vi "Mqtt_Msg_Decode.vi"(8 "error in (no error)":errorcluster, 11 "CMD_Response":string="{\n    \"ID\": \"ac0cc47e-6714-46c6-9d0a-105aa9849fbe\",\n    \"TO\": \"9C6B00576F17\",\n    \"FROM\": \"6805CAB81F91\",\n    \"CMD\": 3,\n    \"CONTENT\": [\n      {\n        \"RACK\": \"101\",\n        \"DUT\": \"1\",\n        \"STATUS\": \"READY\", //READY, MAINTAIN, CLOSE\n        \"REQ_ID\": \"9c67a4e5-71cc-4fd4-b3a2-c356c70535d5\"\n      }\n    ],\n    \"STATUS\": true,\n    \"ERRCODE\": \"\",\n    \"ERRMSG\": \"\",\n    \"TIMESTAMP\": 1757865617\n  }") -> (0 "error out":errorcluster, 3 "Result":T1)   [LabVIEW 2020]
uses:
  <vilib>/addons/JSON API/JSON Value/JSON Value.lvclass
  Ctrl/ReplyCMD0.ctl
  Ctrl/ReplyCMD3.ctl
  Ctrl/ReplyCMD6.ctl
  Ctrl/ReplyCMD9.ctl
  Ctrl/ReplyCMD23.ctl
  Ctrl/ReplyCMD24.ctl
  Ctrl/ReplyCMD25.ctl
  <vilib>/addons/JSON API/JSON Value/Set from JSON string.vi
  <vilib>/addons/JSON API/JSON Value/Get as JSON string.vi
  <vilib>/addons/JSON API/JSON Scalar/Get as U32.vi
  <vilib>/addons/JSON API/JSON Scalar/Get as Boolean.vi
  <vilib>/addons/JSON API/JSON Scalar/Get as Text.vi
  <vilib>/addons/JSON API/JSON Value/Get Array by name.vi
  <vilib>/addons/JSON API/JSON Value/Get Item by name array.vi
  <vilib>/addons/JSON API/Get Polymorphic/JSON GetSet.lvlib
  <vilib>/addons/_JKI.lib/Serialization/JSON/JKI JSON Serialization.lvlib
  <vilib>/addons/JSON API/JSON Scalar/JSON Scalar.lvclass
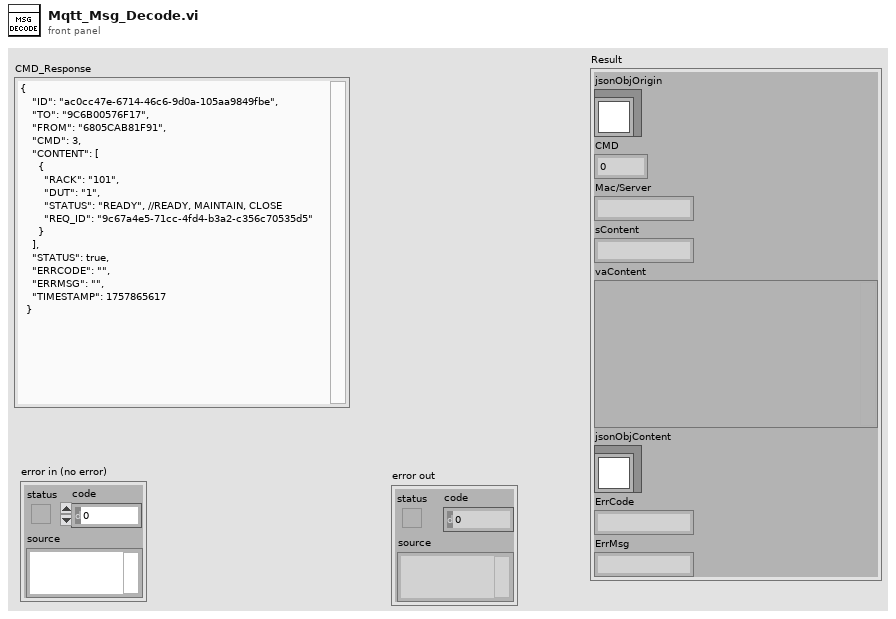
[diagram p1: front panel]
types:
  T1 = cluster{"jsonObjOrigin":refnum<class "JSON Value.lvclass">, "CMD":u32, "Mac/Server":string, "sContent":string, "vaContent":variant, "jsonObjContent":refnum<class "JSON Value.lvclass">, "ErrCode":string, "ErrMsg":string}
  T2 = typedef "ReplyCMD0.ctl" = cluster{"ADD_TOPIC":string}
  T3 = typedef "ReplyCMD3.ctl" = cluster{"RACK":string, "DUT":string, "STATUS":string}
  T4 = typedef "ReplyCMD6.ctl" = cluster{"STATION":string, "RACK":string, "SN":string, "RESULT":string}
  T5 = typedef "ReplyCMD9.ctl" = cluster{"RACK":string, "DUT":string, "CMD":string}
  T6 = typedef "ReplyCMD23.ctl" = cluster{"STATION":string, "RACK":string, "DUT":string, "SN":string, "DESC":string, "RESULT":string, "SET_RACK_STATUS":string}
  T7 = typedef "ReplyCMD24.ctl" = cluster{"STATION":string, "RACK":string, "DUT":string, "SN":string, "MAC_BMC":string, "MAC_SWITCH":string, "MAC_SCM":string}
  T8 = typedef "ReplyCMD25.ctl" = cluster{"STATION":string, "RACK":u32, "DUT":u32}
  T9 = cluster{"H/P":cluster{"Rack#":string, "DUT Status":string[]}[], "F/T-B":cluster{"Rack#":string, "DUT Status":string[]}[], "F/T":cluster{"Rack#":string, "DUT Status":string[]}[]}
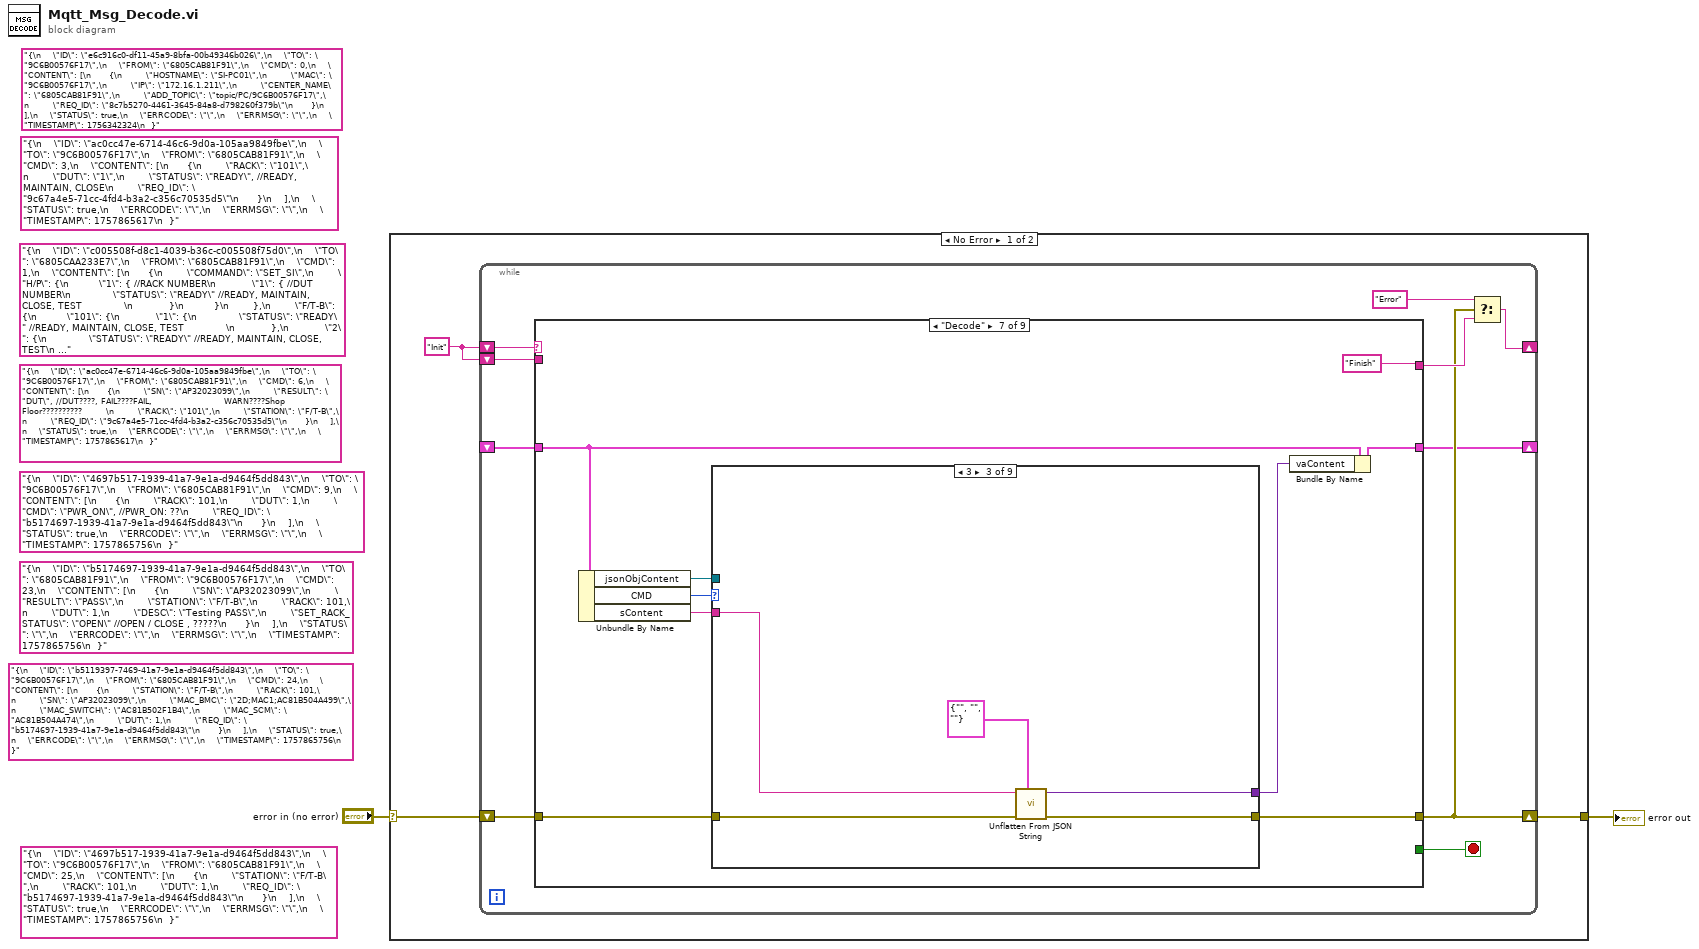
[diagram p0: block diagram]
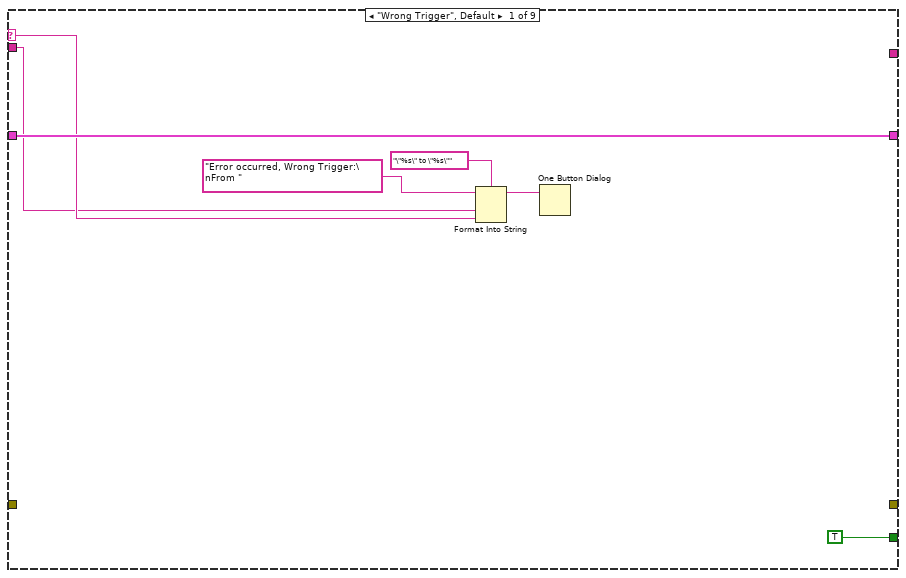
[diagram p2: hidden frame]
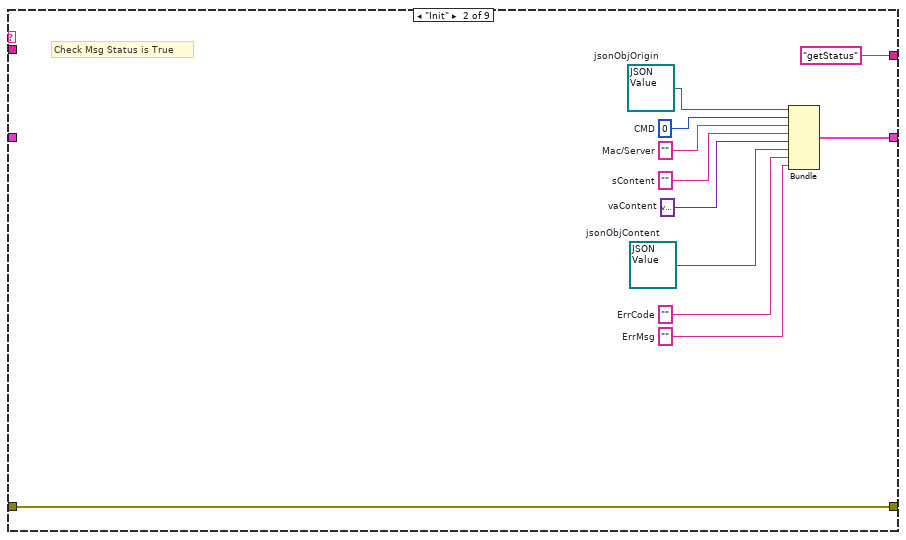
[diagram p3: hidden frame]
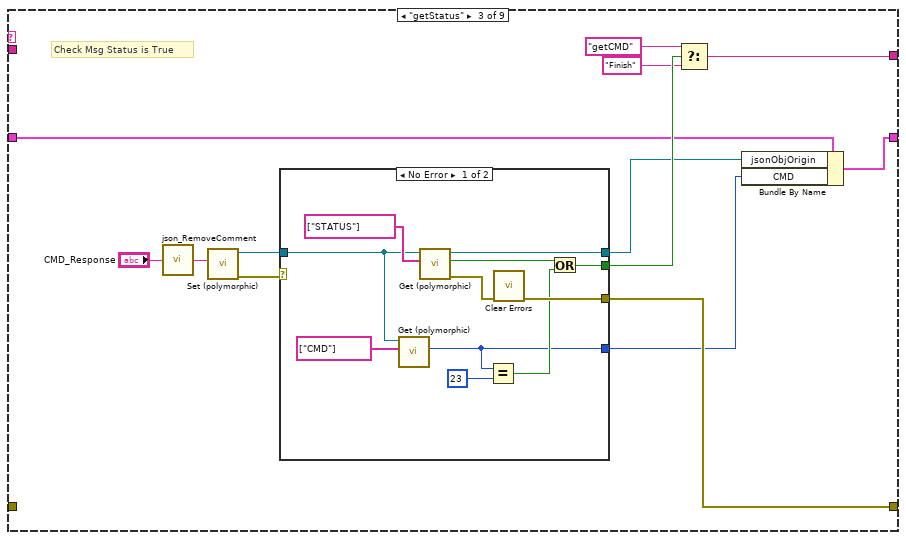
[diagram p4: hidden frame]
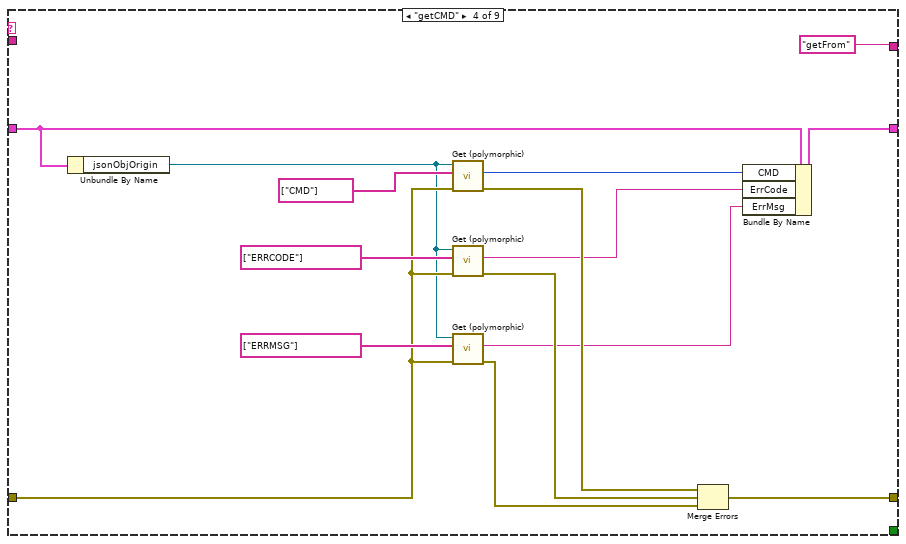
[diagram p6: hidden frame]
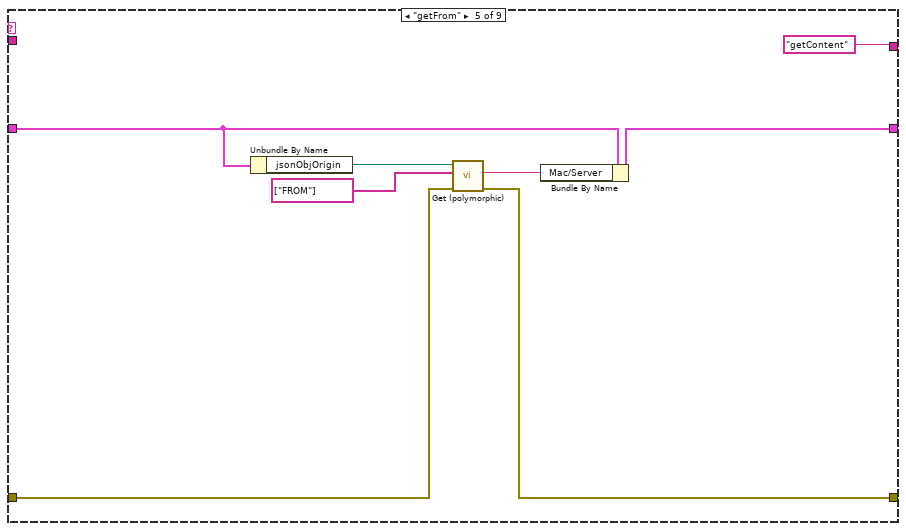
[diagram p7: hidden frame]
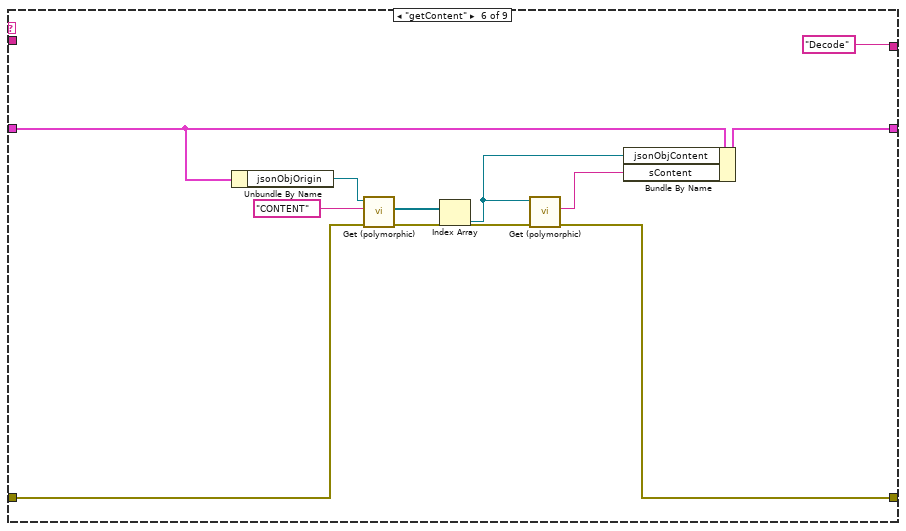
[diagram p8: hidden frame]
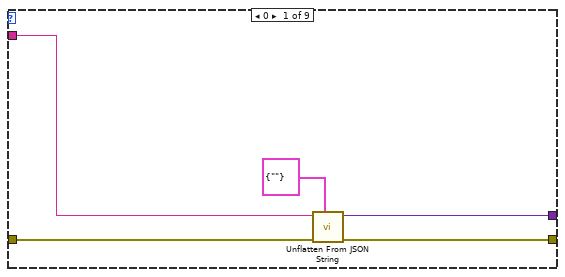
[diagram p9: hidden frame]
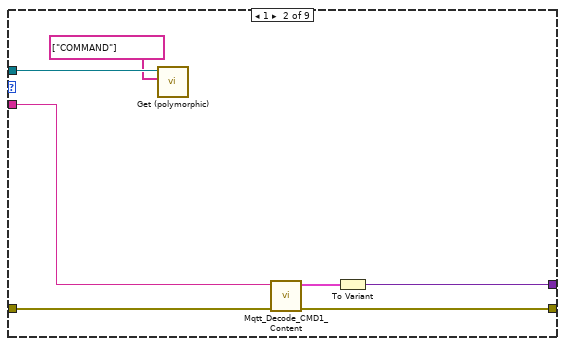
[diagram p10: hidden frame]
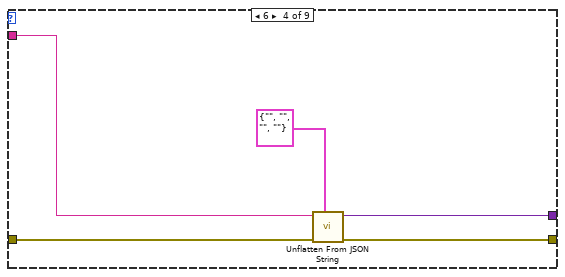
[diagram p11: hidden frame]
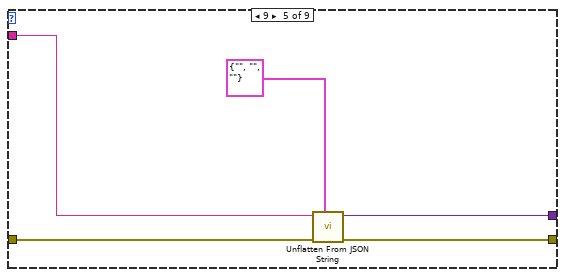
[diagram p12: hidden frame]
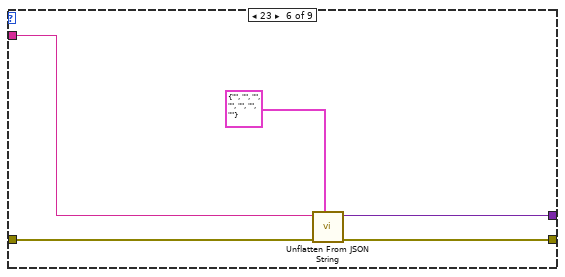
[diagram p13: hidden frame]
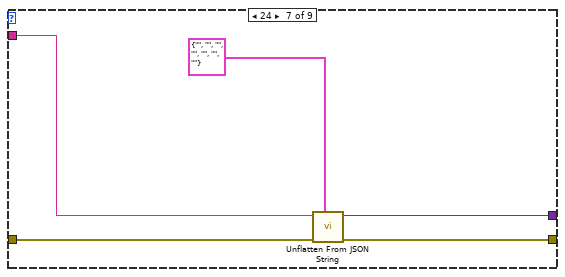
[diagram p14: hidden frame]
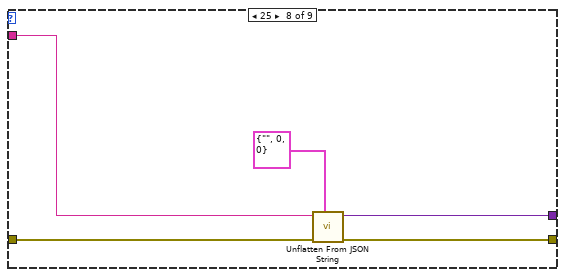
[diagram p15: hidden frame]
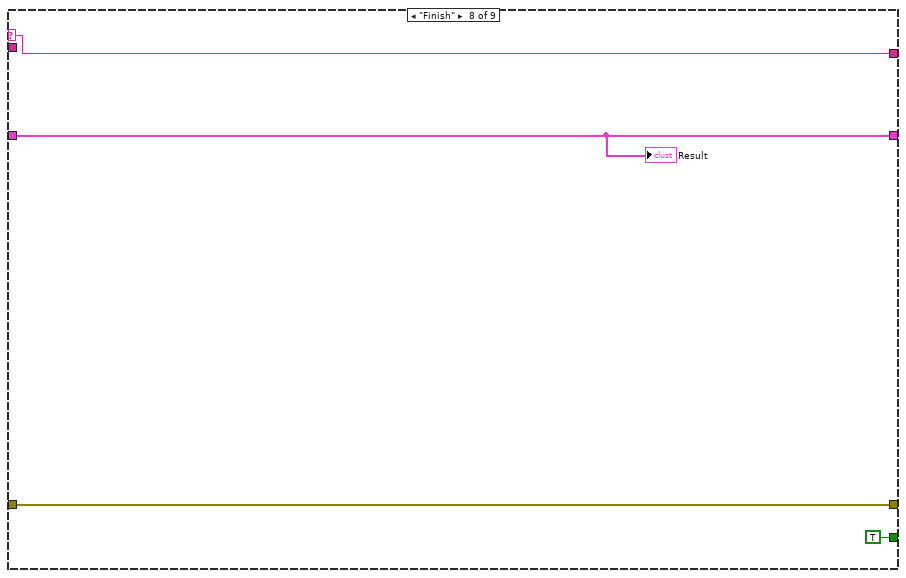
[diagram p17: hidden frame]
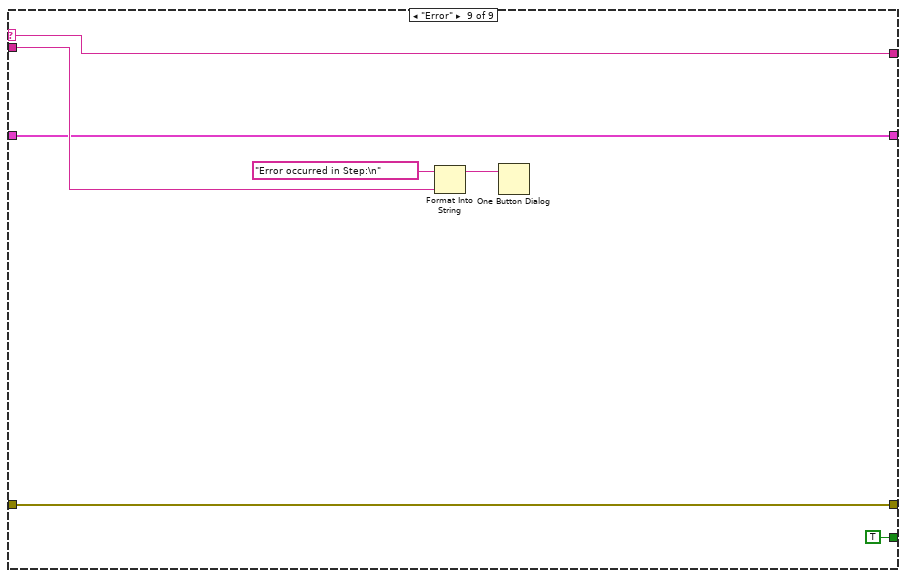
[diagram p18: hidden frame]
diagram:
  (unwired) "{\n    \"ID\": \"b5119397-7469-41a7-9e1a-d9464f5dd843\",\n    \"TO\": \"9C6B00576F17\",\n    \"FROM\": \"6805CAB81F91\",\n    \"CMD\": 24,\n    \"CONTENT\": [\n      {\n        \"STATION\": \"F/T-B\",\n        \"RACK\": 101,\n        \"SN\": \"AP32023099\",\n        \"MAC_BMC\": \"2D;MAC1;AC81B504A499\",\n        \"MAC_SWITCH\": \"AC81B502F1B4\",\n        \"MAC_SCM\": \"AC81B504A474\",\n        \"DUT\": 1,\n        \"REQ_ID\": \"b5174697-1939-41a7-9e1a-d9464f5dd843\"\n      }\n    ],\n    \"STATUS\": true,\n    \"ERRCODE\": \"\",\n    \"ERRMSG\": \"\",\n    \"TIMESTAMP\": 1757865756\n  }" ("CMD_Response")
  (unwired) "{\n    \"ID\": \"b5174697-1939-41a7-9e1a-d9464f5dd843\",\n    \"TO\": \"6805CAB81F91\",\n    \"FROM\": \"9C6B00576F17\",\n    \"CMD\": 23,\n    \"CONTENT\": [\n      {\n        \"SN\": \"AP32023099\",\n        \"RESULT\": \"PASS\",\n        \"STATION\": \"F/T-B\",\n        \"RACK\": 101,\n        \"DUT\": 1,\n        \"DESC\": \"Testing PASS\",\n        \"SET_RACK_STATUS\": \"OPEN\" //OPEN / CLOSE , ?????\n      }\n    ],\n    \"STATUS\": \"\",\n    \"ERRCODE\": \"\",\n    \"ERRMSG\": \"\",\n    \"TIMESTAMP\": 1757865756\n  }" ("CMD_Response")
  (unwired) "{\n    \"ID\": \"4697b517-1939-41a7-9e1a-d9464f5dd843\",\n    \"TO\": \"9C6B00576F17\",\n    \"FROM\": \"6805CAB81F91\",\n    \"CMD\": 9,\n    \"CONTENT\": [\n      {\n        \"RACK\": 101,\n        \"DUT\": 1,\n        \"CMD\": \"PWR_ON\", //PWR_ON: ??\n        \"REQ_ID\": \"b5174697-1939-41a7-9e1a-d9464f5dd843\"\n      }\n    ],\n    \"STATUS\": true,\n    \"ERRCODE\": \"\",\n    \"ERRMSG\": \"\",\n    \"TIMESTAMP\": 1757865756\n  }" ("CMD_Response")
  (unwired) "{\n    \"ID\": \"ac0cc47e-6714-46c6-9d0a-105aa9849fbe\",\n    \"TO\": \"9C6B00576F17\",\n    \"FROM\": \"6805CAB81F91\",\n    \"CMD\": 6,\n    \"CONTENT\": [\n      {\n        \"SN\": \"AP32023099\",\n        \"RESULT\": \"DUT\", //DUT????, FAIL????FAIL,                        WARN????Shop Floor??????????        \n        \"RACK\": \"101\",\n        \"STATION\": \"F/T-B\",\n        \"REQ_ID\": \"9c67a4e5-71cc-4fd4-b3a2-c356c70535d5\"\n      }\n    ],\n    \"STATUS\": true,\n    \"ERRCODE\": \"\",\n    \"ERRMSG\": \"\",\n    \"TIMESTAMP\": 1757865617\n  }" ("CMD_Response")
  (unwired) "{\n    \"ID\": \"c005508f-d8c1-4039-b36c-c005508f75d0\",\n    \"TO\": \"6805CAA233E7\",\n    \"FROM\": \"6805CAB81F91\",\n    \"CMD\": 1,\n    \"CONTENT\": [\n      {\n        \"COMMAND\": \"SET_SI\",\n        \"H/P\": {\n          \"1\": { //RACK NUMBER\n            \"1\": { //DUT NUMBER\n              \"STATUS\": \"READY\" //READY, MAINTAIN, CLOSE, TEST              \n            }\n          }\n        },\n        \"F/T-B\": {\n          \"101\": {\n            \"1\": {\n              \"STATUS\": \"READY\" //READY, MAINTAIN, CLOSE, TEST              \n            },\n            \"2\": {\n              \"STATUS\": \"READY\" //READY, MAINTAIN, CLOSE, TEST\n            },\n            \"3\": {\n              \"STATUS\": \"READY\" //READY, MAINTAIN, CLOSE, TEST\n            },\n            \"4\": {\n              \"STATUS\": \"READY\" //READY, MAINTAIN, CLOSE, TEST\n            },\n            \"5\": {\n              \"STATUS\": \"READY\" //READY, MAINTAIN, CLOSE, TEST\n            }\n          },\n          \"102\": {\n            \"1\": {\n              \"STATUS\": \"READY\" //READY, MAINTAIN, CLOSE, TEST              \n            },\n            \"2\": {\n              \"STATUS\": \"READY\" //READY, MAINTAIN, CLOSE, TEST\n            },\n            \"3\": {\n              \"STATUS\": \"READY\" //READY, MAINTAIN, CLOSE, TEST\n            },\n            \"4\": {\n              \"STATUS\": \"READY\" //READY, MAINTAIN, CLOSE, TEST\n            },\n            \"5\": {\n              \"STATUS\": \"READY\" //READY, MAINTAIN, CLOSE, TEST\n            }\n          },\n          \"103\": {\n            \"1\": {\n              \"STATUS\": \"READY\" //READY, MAINTAIN, CLOSE, TEST              \n            },\n            \"2\": {\n              \"STATUS\": \"READY\" //READY, MAINTAIN, CLOSE, TEST\n            },\n            \"3\": {\n              \"STATUS\": \"READY\" //READY, MAINTAIN, CLOSE, TEST\n            },\n            \"4\": {\n              \"STATUS\": \"READY\" //READY, MAINTAIN, CLOSE, TEST\n            },\n            \"5\": {\n              \"STATUS\": \"READY\" //READY, MAINTAIN, CLOSE, TEST\n            }\n          },\n          \"104\": {\n            \"1\": {\n              \"STATUS\": \"READY\" //READY, MAINTAIN, CLOSE, TEST              \n            },\n            \"2\": {\n              \"STATUS\": \"READY\" //READY, MAINTAIN, CLOSE, TEST\n            },\n            \"3\": {\n              \"STATUS\": \"READY\" //READY, MAINTAIN, CLOSE, TEST\n            },\n            \"4\": {\n              \"STATUS\": \"READY\" //READY, MAINTAIN, CLOSE, TEST\n            },\n            \"5\": {\n              \"STATUS\": \"READY\" //READY, MAINTAIN, CLOSE, TEST\n            }\n          },\n          \"105\": {\n            \"1\": {\n              \"STATUS\": \"READY\" //READY, MAINTAIN, CLOSE, TEST              \n            },\n            \"2\": {\n              \"STATUS\": \"READY\" //READY, MAINTAIN, CLOSE, TEST\n            },\n            \"3\": {\n              \"STATUS\": \"READY\" //READY, MAINTAIN, CLOSE, TEST\n            },\n            \"4\": {\n              \"STATUS\": \"READY\" //READY, MAINTAIN, CLOSE, TEST\n            },\n            \"5\": {\n              \"STATUS\": \"READY\" //READY, MAINTAIN, CLOSE, TEST\n            }\n          },\n          \"106\": {\n            \"1\": {\n              \"STATUS\": \"READY\" //READY, MAINTAIN, CLOSE, TEST              \n            },\n            \"2\": {\n              \"STATUS\": \"READY\" //READY, MAINTAIN, CLOSE, TEST\n            },\n            \"3\": {\n              \"STATUS\": \"READY\" //READY, MAINTAIN, CLOSE, TEST\n            },\n            \"4\": {\n              \"STATUS\": \"READY\" //READY, MAINTAIN, CLOSE, TEST\n            },\n            \"5\": {\n              \"STATUS\": \"READY\" //READY, MAINTAIN, CLOSE, TEST\n            }\n          },\n          \"107\": {\n            \"1\": {\n              \"STATUS\": \"READY\" //READY, MAINTAIN, CLOSE, TEST              \n            },\n            \"2\": {\n              \"STATUS\": \"READY\" //READY, MAINTAIN, CLOSE, TEST\n            },\n            \"3\": {\n              \"STATUS\": \"READY\" //READY, MAINTAIN, CLOSE, TEST\n            },\n            \"4\": {\n              \"STATUS\": \"READY\" //READY, MAINTAIN, CLOSE, TEST\n            },\n            \"5\": {\n              \"STATUS\": \"READY\" //READY, MAINTAIN, CLOSE, TEST\n            }\n          },\n          \"108\": {\n            \"1\": {\n              \"STATUS\": \"READY\" //READY, MAINTAIN, CLOSE, TEST              \n            },\n            \"2\": {\n              \"STATUS\": \"READY\" //READY, MAINTAIN, CLOSE, TEST\n            },\n            \"3\": {\n              \"STATUS\": \"READY\" //READY, MAINTAIN, CLOSE, TEST\n            },\n            \"4\": {\n              \"STATUS\": \"READY\" //READY, MAINTAIN, CLOSE, TEST\n            },\n            \"5\": {\n              \"STATUS\": \"READY\" //READY, MAINTAIN, CLOSE, TEST\n            }\n          },\n          \"109\": {\n            \"1\": {\n              \"STATUS\": \"READY\" //READY, MAINTAIN, CLOSE, TEST              \n            },\n            \"2\": {\n              \"STATUS\": \"READY\" //READY, MAINTAIN, CLOSE, TEST\n            },\n            \"3\": {\n              \"STATUS\": \"READY\" //READY, MAINTAIN, CLOSE, TEST\n            },\n            \"4\": {\n              \"STATUS\": \"READY\" //READY, MAINTAIN, CLOSE, TEST\n            },\n            \"5\": {\n              \"STATUS\": \"READY\" //READY, MAINTAIN, CLOSE, TEST\n            }\n          },\n          \"110\": {\n            \"1\": {\n              \"STATUS\": \"READY\" //READY, MAINTAIN, CLOSE, TEST              \n            },\n            \"2\": {\n              \"STATUS\": \"READY\" //READY, MAINTAIN, CLOSE, TEST\n            },\n            \"3\": {\n              \"STATUS\": \"READY\" //READY, MAINTAIN, CLOSE, TEST\n            },\n            \"4\": {\n              \"STATUS\": \"READY\" //READY, MAINTAIN, CLOSE, TEST\n            },\n            \"5\": {\n              \"STATUS\": \"READY\" //READY, MAINTAIN, CLOSE, TEST\n            }\n          },\n          \"111\": {\n            \"1\": {\n              \"STATUS\": \"READY\" //READY, MAINTAIN, CLOSE, TEST              \n            },\n            \"2\": {\n              \"STATUS\": \"READY\" //READY, MAINTAIN, CLOSE, TEST\n            },\n            \"3\": {\n              \"STATUS\": \"READY\" //READY, MAINTAIN, CLOSE, TEST\n            },\n            \"4\": {\n              \"STATUS\": \"READY\" //READY, MAINTAIN, CLOSE, TEST\n            },\n            \"5\": {\n              \"STATUS\": \"READY\" //READY, MAINTAIN, CLOSE, TEST\n            }\n          },\n          \"112\": {\n            \"1\": {\n              \"STATUS\": \"READY\" //READY, MAINTAIN, CLOSE, TEST              \n            },\n            \"2\": {\n              \"STATUS\": \"READY\" //READY, MAINTAIN, CLOSE, TEST\n            },\n            \"3\": {\n              \"STATUS\": \"READY\" //READY, MAINTAIN, CLOSE, TEST\n            },\n            \"4\": {\n              \"STATUS\": \"READY\" //READY, MAINTAIN, CLOSE, TEST\n            },\n            \"5\": {\n              \"STATUS\": \"READY\" //READY, MAINTAIN, CLOSE, TEST\n            }\n          }\n        },\n        \"F/T\": {\n          \"201\": {\n            \"1\": {\n              \"STATUS\": \"READY\" //READY, MAINTAIN, CLOSE, TEST              \n            },\n            \"2\": {\n              \"STATUS\": \"READY\" //READY, MAINTAIN, CLOSE, TEST\n            },\n            \"3\": {\n              \"STATUS\": \"READY\" //READY, MAINTAIN, CLOSE, TEST\n            },\n            \"4\": {\n              \"STATUS\": \"READY\" //READY, MAINTAIN, CLOSE, TEST\n            },\n            \"5\": {\n              \"STATUS\": \"READY\" //READY, MAINTAIN, CLOSE, TEST\n            }\n          },\n          \"202\": {\n            \"1\": {\n              \"STATUS\": \"READY\" //READY, MAINTAIN, CLOSE, TEST              \n            },\n            \"2\": {\n              \"STATUS\": \"READY\" //READY, MAINTAIN, CLOSE, TEST\n            },\n            \"3\": {\n              \"STATUS\": \"READY\" //READY, MAINTAIN, CLOSE, TEST\n            },\n            \"4\": {\n              \"STATUS\": \"READY\" //READY, MAINTAIN, CLOSE, TEST\n            },\n            \"5\": {\n              \"STATUS\": \"READY\" //READY, MAINTAIN, CLOSE, TEST\n            }\n          },\n          \"203\": {\n            \"1\": {\n              \"STATUS\": \"READY\" //READY, MAINTAIN, CLOSE, TEST              \n            },\n            \"2\": {\n              \"STATUS\": \"READY\" //READY, MAINTAIN, CLOSE, TEST\n            },\n            \"3\": {\n              \"STATUS\": \"READY\" //READY, MAINTAIN, CLOSE, TEST\n            },\n            \"4\": {\n              \"STATUS\": \"READY\" //READY, MAINTAIN, CLOSE, TEST\n            },\n            \"5\": {\n              \"STATUS\": \"READY\" //READY, MAINTAIN, CLOSE, TEST\n            }\n          },\n          \"204\": {\n            \"1\": {\n              \"STATUS\": \"READY\" //READY, MAINTAIN, CLOSE, TEST              \n            },\n            \"2\": {\n              \"STATUS\": \"READY\" //READY, MAINTAIN, CLOSE, TEST\n            },\n            \"3\": {\n              \"STATUS\": \"READY\" //READY, MAINTAIN, CLOSE, TEST\n            },\n            \"4\": {\n              \"STATUS\": \"READY\" //READY, MAINTAIN, CLOSE, TEST\n            },\n            \"5\": {\n              \"STATUS\": \"READY\" //READY, MAINTAIN, CLOSE, TEST\n            }\n          },\n          \"205\": {\n            \"1\": {\n              \"STATUS\": \"READY\" //READY, MAINTAIN, CLOSE, TEST              \n            },\n            \"2\": {\n              \"STATUS\": \"READY\" //READY, MAINTAIN, CLOSE, TEST\n            },\n            \"3\": {\n              \"STATUS\": \"READY\" //READY, MAINTAIN, CLOSE, TEST\n            },\n            \"4\": {\n              \"STATUS\": \"READY\" //READY, MAINTAIN, CLOSE, TEST\n            },\n            \"5\": {\n              \"STATUS\": \"READY\" //READY, MAINTAIN, CLOSE, TEST\n            }\n          },\n          \"206\": {\n            \"1\": {\n              \"STATUS\": \"READY\" //READY, MAINTAIN, CLOSE, TEST              \n            },\n            \"2\": {\n              \"STATUS\": \"READY\" //READY, MAINTAIN, CLOSE, TEST\n            },\n            \"3\": {\n              \"STATUS\": \"READY\" //READY, MAINTAIN, CLOSE, TEST\n            },\n            \"4\": {\n              \"STATUS\": \"READY\" //READY, MAINTAIN, CLOSE, TEST\n            },\n            \"5\": {\n              \"STATUS\": \"READY\" //READY, MAINTAIN, CLOSE, TEST\n            }\n          },\n          \"207\": {\n            \"1\": {\n              \"STATUS\": \"READY\" //READY, MAINTAIN, CLOSE, TEST              \n            },\n            \"2\": {\n              \"STATUS\": \"READY\" //READY, MAINTAIN, CLOSE, TEST\n            },\n            \"3\": {\n              \"STATUS\": \"READY\" //READY, MAINTAIN, CLOSE, TEST\n            },\n            \"4\": {\n              \"STATUS\": \"READY\" //READY, MAINTAIN, CLOSE, TEST\n            },\n            \"5\": {\n              \"STATUS\": \"READY\" //READY, MAINTAIN, CLOSE, TEST\n            }\n          },\n          \"208\": {\n            \"1\": {\n              \"STATUS\": \"READY\" //READY, MAINTAIN, CLOSE, TEST              \n            },\n            \"2\": {\n              \"STATUS\": \"READY\" //READY, MAINTAIN, CLOSE, TEST\n            },\n            \"3\": {\n              \"STATUS\": \"READY\" //READY, MAINTAIN, CLOSE, TEST\n            },\n            \"4\": {\n              \"STATUS\": \"READY\" //READY, MAINTAIN, CLOSE, TEST\n            },\n            \"5\": {\n              \"STATUS\": \"READY\" //READY, MAINTAIN, CLOSE, TEST\n            }\n          },\n          \"209\": {\n            \"1\": {\n              \"STATUS\": \"READY\" //READY, MAINTAIN, CLOSE, TEST              \n            },\n            \"2\": {\n              \"STATUS\": \"READY\" //READY, MAINTAIN, CLOSE, TEST\n            },\n            \"3\": {\n              \"STATUS\": \"READY\" //READY, MAINTAIN, CLOSE, TEST\n            },\n            \"4\": {\n              \"STATUS\": \"READY\" //READY, MAINTAIN, CLOSE, TEST\n            },\n            \"5\": {\n              \"STATUS\": \"READY\" //READY, MAINTAIN, CLOSE, TEST\n            }\n          },\n          \"210\": {\n            \"1\": {\n              \"STATUS\": \"READY\" //READY, MAINTAIN, CLOSE, TEST              \n            },\n            \"2\": {\n              \"STATUS\": \"READY\" //READY, MAINTAIN, CLOSE, TEST\n            },\n            \"3\": {\n              \"STATUS\": \"READY\" //READY, MAINTAIN, CLOSE, TEST\n            },\n            \"4\": {\n              \"STATUS\": \"READY\" //READY, MAINTAIN, CLOSE, TEST\n            },\n            \"5\": {\n              \"STATUS\": \"READY\" //READY, MAINTAIN, CLOSE, TEST\n            }\n          },\n          \"211\": {\n            \"1\": {\n              \"STATUS\": \"READY\" //READY, MAINTAIN, CLOSE, TEST              \n            },\n            \"2\": {\n              \"STATUS\": \"READY\" //READY, MAINTAIN, CLOSE, TEST\n            },\n            \"3\": {\n              \"STATUS\": \"READY\" //READY, MAINTAIN, CLOSE, TEST\n            },\n            \"4\": {\n              \"STATUS\": \"READY\" //READY, MAINTAIN, CLOSE, TEST\n            },\n            \"5\": {\n              \"STATUS\": \"READY\" //READY, MAINTAIN, CLOSE, TEST\n            }\n          },\n          \"212\": {\n            \"1\": {\n              \"STATUS\": \"READY\" //READY, MAINTAIN, CLOSE, TEST              \n            },\n            \"2\": {\n              \"STATUS\": \"READY\" //READY, MAINTAIN, CLOSE, TEST\n            },\n            \"3\": {\n              \"STATUS\": \"READY\" //READY, MAINTAIN, CLOSE, TEST\n            },\n            \"4\": {\n              \"STATUS\": \"READY\" //READY, MAINTAIN, CLOSE, TEST\n            },\n            \"5\": {\n              \"STATUS\": \"READY\" //READY, MAINTAIN, CLOSE, TEST\n            }\n          }\n        },\n        \"REQ_ID\": \"c005508f-d8c1-4039-b36c-d37dd9f875d0\"\n      }\n    ],\n    \"STATUS\": true,\n    \"ERRCODE\": \"\",\n    \"ERRMSG\": \"\",\n    \"TIMESTAMP\": 1758590005\n  }"
  (unwired) "{\n    \"ID\": \"e6c916c0-df11-45a9-8bfa-00b49346b026\",\n    \"TO\": \"9C6B00576F17\",\n    \"FROM\": \"6805CAB81F91\",\n    \"CMD\": 0,\n    \"CONTENT\": [\n      {\n        \"HOSTNAME\": \"SI-PC01\",\n        \"MAC\": \"9C6B00576F17\",\n        \"IP\": \"172.16.1.211\",\n        \"CENTER_NAME\": \"6805CAB81F91\",\n        \"ADD_TOPIC\": \"topic/PC/9C6B00576F17\",\n        \"REQ_ID\": \"8c7b5270-4461-3645-84a8-d798260f379b\"\n      }\n    ],\n    \"STATUS\": true,\n    \"ERRCODE\": \"\",\n    \"ERRMSG\": \"\",\n    \"TIMESTAMP\": 1756342324\n  }" ("CMD_Response")
  (unwired) "{\n    \"ID\": \"4697b517-1939-41a7-9e1a-d9464f5dd843\",\n    \"TO\": \"9C6B00576F17\",\n    \"FROM\": \"6805CAB81F91\",\n    \"CMD\": 25,\n    \"CONTENT\": [\n      {\n        \"STATION\": \"F/T-B\",\n        \"RACK\": 101,\n        \"DUT\": 1,\n        \"REQ_ID\": \"b5174697-1939-41a7-9e1a-d9464f5dd843\"\n      }\n    ],\n    \"STATUS\": true,\n    \"ERRCODE\": \"\",\n    \"ERRMSG\": \"\",\n    \"TIMESTAMP\": 1757865756\n  }" ("CMD_Response")
  (unwired) "{\n    \"ID\": \"ac0cc47e-6714-46c6-9d0a-105aa9849fbe\",\n    \"TO\": \"9C6B00576F17\",\n    \"FROM\": \"6805CAB81F91\",\n    \"CMD\": 3,\n    \"CONTENT\": [\n      {\n        \"RACK\": \"101\",\n        \"DUT\": \"1\",\n        \"STATUS\": \"READY\", //READY, MAINTAIN, CLOSE\n        \"REQ_ID\": \"9c67a4e5-71cc-4fd4-b3a2-c356c70535d5\"\n      }\n    ],\n    \"STATUS\": true,\n    \"ERRCODE\": \"\",\n    \"ERRMSG\": \"\",\n    \"TIMESTAMP\": 1757865617\n  }" ("CMD_Response")
  n1 = case shown="No Error" "error in (no error)" {
    selector: "error in (no error)" -> [w4 w157]
    tunnel: [w3 w157] -> w2
    frame No Error {
      w5 = "Init"
      n2 = while {
        shift-right: [w13] -> _
        shift-left: w5 -> [w15]
        shift-left: w5 -> [w11]
        shift-right: [w9] -> w3
        shift-left: w4 -> [w10]
        shift-right: [w7] -> _
        shift-left: _ -> [w6]
        stop <- w8 stop-if-true
        n3 = case shown="\"Decode\"" w15 {
          selector: w15 -> [w17 _ _ _ _ _ _ w149 w153]
          tunnel: [_ w26 w41 w68 w76 w86 w97 w148 w152] -> w9
          tunnel: [_ "getStatus" w38 "getFrom" ("t") "getContent" ("t") "Decode" ("t") "Finish" ("t") w149 w153] -> w14
          tunnel: w11 -> [w16 _ _ _ _ _ _ _ w156]
          tunnel: w10 -> [_ w26 _ w63 w75 w88 w98 w148 w152]
          tunnel: [TRUE _ _ _ _ _ _ TRUE TRUE] -> w8
          tunnel: [w19 w33 w36 w72 w79 w92 w96 w146 w150] -> w7
          tunnel: w6 -> [w19 _ w37 w74 w82 w93 w102 w146 w150]
          frame "Wrong Trigger", Default {
            n4 = Format Into String(format string="\"%s\" to \"%s\"", initial string="Error occurred, Wrong Trigger:\nFrom ", w16, w17) -> (resulting string=w22:string)  [unwired: 1 in, 1 out]
            n5 = One Button Dialog(message=w22) -> ()  [unwired: 1 in, 1 out]
          }
          frame "Init" {
            w23 = ""  # ErrMsg
            w24 = ""  # ErrCode
            w25 = refnum<class "JSON Value.lvclass"> refnum  # jsonObjContent
            w28 = refnum<class "JSON Value.lvclass"> refnum  # jsonObjOrigin
            w29 = ""  # Mac/Server
            w30 = variant  # vaContent
            w31 = ""  # sContent
            w32 = u32 0  # CMD
            # "Check Msg Status is True"
            n6 = Bundle("jsonObjOrigin"=w28, "CMD"=w32, "Mac/Server"=w29, "sContent"=w31, "vaContent"=w30, "jsonObjContent"=w25, "ErrCode"=w24, "ErrMsg"=w23) -> (w33:T1)  [unwired: 1 in]
          }
          frame "getStatus" {
            # "Check Msg Status is True"
            n7 = call "json_RemoveComment.vi"("json with comment"="CMD_Response") -> ("json without comment"=w45:string)
            n8 = call-poly <vilib>:"Set (polymorphic).vi"("JSON stream"=w45) -> ("error out"=w43:errorcluster, "JSON Value out"=w44:refnum<class "JSON Value.lvclass">)  [unwired: 8 in, 1 out]
            n9 = case shown="No Error" w43 {
              selector: w43 -> [_ w58]
              tunnel: w44 -> [w51 w59]
              tunnel: [w49 _] -> w42
              tunnel: [w54 w59] -> w35
              tunnel: [w53 w58] -> w41
              tunnel: [w47 _] -> w34
              frame No Error {
                n10 = call-poly <vilib>:"Get (polymorphic).vi"("Name Array"=string[] ["CMD"], "JSON Scalar in"=w51) -> ("Number"=w47:u32)  [unwired: 7 in, 2 out]
                n11 = call-poly <vilib>:"Get (polymorphic).vi"("Name Array"=string[] ["STATUS"], "JSON Value in"=w51) -> ("error out"=w56:errorcluster, "Boolean"=w55:bool, "JSON Value out"=w54:refnum<class "JSON Value.lvclass">)  [unwired: 7 in]
                n12 = Equal?(x=w47, y=u32 23) -> (x = y?=w48:bool)
                n13 = call <vilib>:"Clear Errors.vi"("error in (no error)"=w56) -> ("error out"=w53:errorcluster)  [unwired: 5 in, 1 out]
                n14 = Or(x=w55, y=w48) -> (x .or. y?=w49:bool)
              }
              frame Error {
              }
            }
            n15 = Select(t="getCMD", s=w42, f="Finish") -> (s? t:f=w38:string)
            n16 = Bundle By Name(cluster=w37, "jsonObjOrigin"=w35, "CMD"=w34) -> (w36:T1)
          }
          frame "getCMD" {
            n17 = Unbundle By Name(w74) -> ("jsonObjOrigin"=w62:refnum<class "JSON Value.lvclass">)
            n18 = call-poly <vilib>:"Get (polymorphic).vi"("error in (no error)"=w63, "Name Array"=string[] ["CMD"], "JSON Scalar in"=w62) -> ("error out"=w69:errorcluster, "Number"=w71:u32)  [unwired: 6 in, 1 out]
            n19 = call-poly <vilib>:"Get (polymorphic).vi"("error in (no error)"=w63, "Name Array"=string[] ["ERRCODE"], "JSON Scalar in"=w62) -> ("error out"=w66:errorcluster, "LabVIEW Text"=w61:string)  [unwired: 6 in, 1 out]
            n20 = call-poly <vilib>:"Get (polymorphic).vi"("error in (no error)"=w63, "Name Array"=string[] ["ERRMSG"], "JSON Scalar in"=w62) -> ("error out"=w67:errorcluster, "LabVIEW Text"=w60:string)  [unwired: 6 in, 1 out]
            n21 = Merge Errors(w69, w66, w67) -> (w68:errorcluster)
            n22 = Bundle By Name(cluster=w74, "CMD"=w71, "ErrCode"=w61, "ErrMsg"=w60) -> (w72:T1)
          }
          frame "getFrom" {
            n23 = Unbundle By Name(w82) -> ("jsonObjOrigin"=w81:refnum<class "JSON Value.lvclass">)
            n24 = call-poly <vilib>:"Get (polymorphic).vi"("error in (no error)"=w75, "Name Array"=string[] ["FROM"], "JSON Scalar in"=w81) -> ("error out"=w76:errorcluster, "LabVIEW Text"=w78:string)  [unwired: 6 in, 1 out]
            n25 = Bundle By Name(cluster=w82, "Mac/Server"=w78) -> (w79:T1)
          }
          frame "getContent" {
            n26 = Unbundle By Name(w93) -> ("jsonObjOrigin"=w87:refnum<class "JSON Value.lvclass">)
            n27 = call-poly <vilib>:"Get (polymorphic).vi"("error in (no error)"=w88, "name"="CONTENT", "JSON Value In"=w87) -> ("error out"=w90:errorcluster, "Array"=w84:refnum<class "JSON Value.lvclass">[])  [unwired: 5 in, 2 out]
            n28 = Index Array(array=w84) -> (element=w83:refnum<class "JSON Value.lvclass">)  [unwired: 1 in]
            n29 = call-poly <vilib>:"Get (polymorphic).vi"("error in (no error)"=w90, "JSON Value in"=w83) -> ("error out"=w86:errorcluster, "<JSON>"=w85:string)  [unwired: 8 in]
            n30 = Bundle By Name(cluster=w93, "jsonObjContent"=w83, "sContent"=w85) -> (w92:T1)
          }
          frame "Decode" {
            n31 = Unbundle By Name(w102) -> ("jsonObjContent"=w94:refnum<class "JSON Value.lvclass">, "CMD"=w100:u32, "sContent"=w99:string)
            n32 = case shown="3" w100 {
              tunnel: w99 -> [w107 w112 w119 w124 w129 w134 w139 w144 _]
              tunnel: w98 -> [w106 w111 w118 w123 w128 w133 w138 w143 w145]
              tunnel: [w105 w110 w117 w122 w127 w132 w137 w142 w145] -> w97
              tunnel: [w104 w108 w116 w121 w126 w131 w136 w141 _] -> w95
              tunnel: w94 -> [_ w114 _ _ _ _ _ _ _]
              frame 0 {
                n33 = call <vilib>:"Unflatten From JSON String.vi"("Type and Defaults"=T2 {"ADD_TOPIC"=""}, "error in"=w106, "JSON String"=w107) -> ("error out"=w105:errorcluster, "Variant"=w104:variant)  [unwired: 7 in]
              }
              frame 1 {
                n34 = call-poly <vilib>:"Get (polymorphic).vi"("Name Array"=string[] ["COMMAND"], "JSON Scalar in"=w114) -> ()  [unwired: 7 in, 3 out]
                n35 = call "Mqtt_Decode_CMD1_Content.vi"("error in (no error)"=w111, "jsContent"=w112) -> ("error out"=w110:errorcluster, "clusterContent"=w109:T9)  [unwired: 8 in]
                n36 = To Variant(anything=w109) -> (Variant=w108:variant)
              }
              frame 3 {
                n37 = call <vilib>:"Unflatten From JSON String.vi"("Type and Defaults"=T3 {"RACK"="", "DUT"="", "STATUS"=""}, "error in"=w118, "JSON String"=w119) -> ("error out"=w117:errorcluster, "Variant"=w116:variant)  [unwired: 7 in]
              }
              frame 6 {
                n38 = call <vilib>:"Unflatten From JSON String.vi"("Type and Defaults"=T4 {"STATION"="", "RACK"="", "SN"="", "RESULT"=""}, "error in"=w123, "JSON String"=w124) -> ("error out"=w122:errorcluster, "Variant"=w121:variant)  [unwired: 7 in]
              }
              frame 9 {
                n39 = call <vilib>:"Unflatten From JSON String.vi"("Type and Defaults"=T5 {"RACK"="", "DUT"="", "CMD"=""}, "error in"=w128, "JSON String"=w129) -> ("error out"=w127:errorcluster, "Variant"=w126:variant)  [unwired: 7 in]
              }
              frame 23 {
                n40 = call <vilib>:"Unflatten From JSON String.vi"("Type and Defaults"=T6 {"STATION"="", "RACK"="", "DUT"="", "SN"="", "DESC"="", "RESULT"="", "SET_RACK_STATUS"=""}, "error in"=w133, "JSON String"=w134) -> ("error out"=w132:errorcluster, "Variant"=w131:variant)  [unwired: 7 in]
              }
              frame 24 {
                n41 = call <vilib>:"Unflatten From JSON String.vi"("Type and Defaults"=T7 {"STATION"="", "RACK"="", "DUT"="", "SN"="", "MAC_BMC"="", "MAC_SWITCH"="", "MAC_SCM"=""}, "error in"=w138, "JSON String"=w139) -> ("error out"=w137:errorcluster, "Variant"=w136:variant)  [unwired: 7 in]
              }
              frame 25 {
                n42 = call <vilib>:"Unflatten From JSON String.vi"("Type and Defaults"=T8 {"STATION"="", "RACK"=0, "DUT"=0}, "error in"=w143, "JSON String"=w144) -> ("error out"=w142:errorcluster, "Variant"=w141:variant)  [unwired: 7 in]
              }
              frame Default {
              }
            }
            n43 = Bundle By Name(cluster=w102, "vaContent"=w95) -> (w96:T1)
          }
          frame "Finish" {
            "Result" <- w146
          }
          frame "Error" {
            n44 = Format Into String(initial string="Error occurred in Step:\n", w156) -> (resulting string=w154:string)  [unwired: 2 in, 1 out]
            n45 = One Button Dialog(message=w154) -> ()  [unwired: 1 in, 1 out]
          }
        }
        n46 = Select(t="Error", s=w9, f=w14) -> (s? t:f=w13:string)
      }
    }
    frame Error {
    }
  }
  "error out" <- w2
